vi "Release Exclusive Access.vi"(0 "semaphore":T1, 2 "error in (no error)":errorcluster) -> (7 "error out":errorcluster)   [LabVIEW 2018, in "3458A Virtual Digitizer.lvlib" / "3458A Digitizing Low Levels.lvlib"]
doc: "Releases exclusive access using the semaphore. It is used to ensure only one instance of this driver accesses the bus at thse same time. \nIf the named semaphore is not found, it ignores the error. The sempahore must be created first! Call this whenever exclusive acces section ends otherwise other instances of this driver may get locked!"
uses:
  3458A Digitizing Low Levels.lvlib
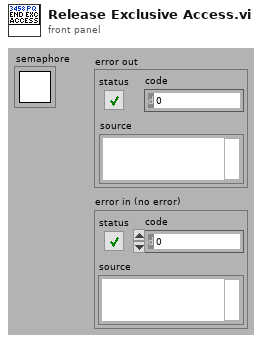
[diagram p1: front panel]
types:
  T1 = typedef "Semaphore RefNum" = refnum<k1>
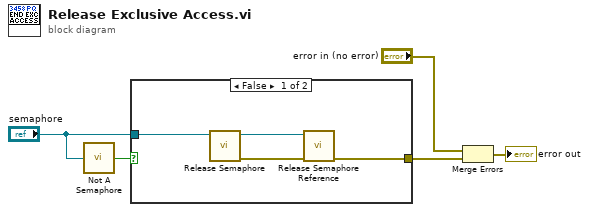
[diagram p0: block diagram]
diagram:
  n1 = call <vilib>:"Not A Semaphore.vi"("semaphore"="semaphore") -> ("not a semaphore"=w1:bool)
  n2 = case shown="False" w1 {
    tunnel: "semaphore" -> [w8 _]
    tunnel: [w9 _] -> w5
    frame False {
      n3 = call <vilib>:"Release Semaphore.vi"("semaphore"=w8) -> ("error out"=w7:errorcluster, "semaphore out"=w6:T1)  [unwired: 5 in]
      n4 = call <vilib>:"Release Semaphore Reference.vi"("error in (no error)"=w7, "semaphore"=w6) -> ("error out"=w9:errorcluster)  [unwired: 8 in, 1 out]
    }
    frame True {
    }
  }
  n5 = Merge Errors("error in (no error)", w5) -> (→"error out":errorcluster)
